vi "UI_AutoRefresh_Init.vi"(8 "error in (no error)":errorcluster, 10 "Parameters":T1={"Write TipStrips with details (T)"=TRUE, "Write Captions with UserLabels (T)"=TRUE, "Mode (ind only)"=enum."Indicators only"}, 11 "UI_Actor in":refnum<class "UI_Actor.lvclass">) -> (0 "error out":errorcluster, 3 "UI_Actor out":refnum<class "UI_Actor.lvclass">)   [LabVIEW 2020, in "UI_Actor.lvlib" / "UI_Actor.lvclass"]
uses:
  UI_Actor.lvclass
  ctl_AR_Parameters.ctl
  ctl_AR_Mode.ctl
  ctl_AR_Elmt.ctl
  UI_Actor.lvclass/UI_Actor.ctl
  UI_Actor Messages/UI_AutoRefresh_Init Msg/UI_AutoRefresh_Init Msg.lvclass/UI_AutoRefresh_Init Msg.ctl
  support/Actor Framework.lvlibp/1abvi3w/vi.lib/ActorFramework/Message Enqueuer/Enqueue.vi
  support/Databox.lvlibp/TypesTools/Config/Read System Label.vi
  UI_Actor Messages/UI_AutoRefresh_Init Msg/UI_AutoRefresh_Init Msg.lvclass
  support/Databox.lvlibp/TypesTools/Config/Config.lvclass
  support/Databox.lvlibp/TypesTools/Data/Data.lvclass
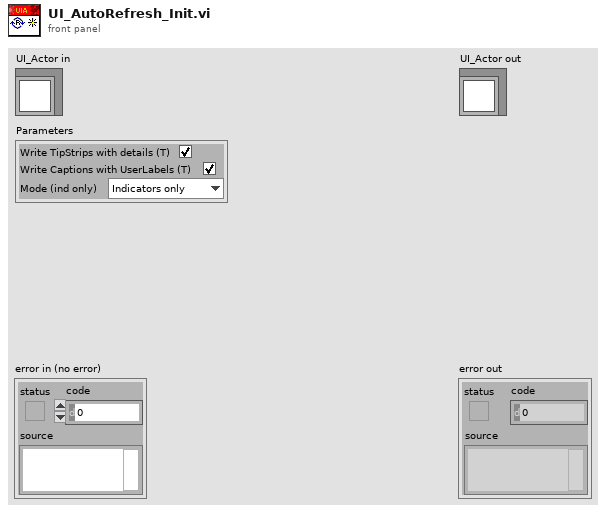
[diagram p1: front panel]
types:
  T1 = typedef "UI_Actor.lvlib/UI_Actor.lvclass/ctl_AR_Parameters.ctl" = cluster{"Write TipStrips with details (T)":bool, "Write Captions with UserLabels (T)":bool, "Mode (ind only)":T2}
  T2 = typedef "UI_Actor.lvlib/UI_Actor.lvclass/ctl_AR_Mode.ctl" = enum16{"Controls only", "Indicators only", "All"}
  T3 = typedef "UI_Actor.lvlib/UI_Actor.lvclass/ctl_AR_Elmt.ctl" = cluster{"AR by Index":bool, "Ref":refnum<vi>, "Index":i32, "Class ID":u32, "Sourcer":string, "SysLab":string}
  T4 = typedef "UI_Actor.lvlib/UI_Actor.lvclass/ctl_InternalMapItem.ctl" = cluster{"Config":refnum<class "Config.lvclass">, "LatestData":refnum<class "Data.lvclass">}
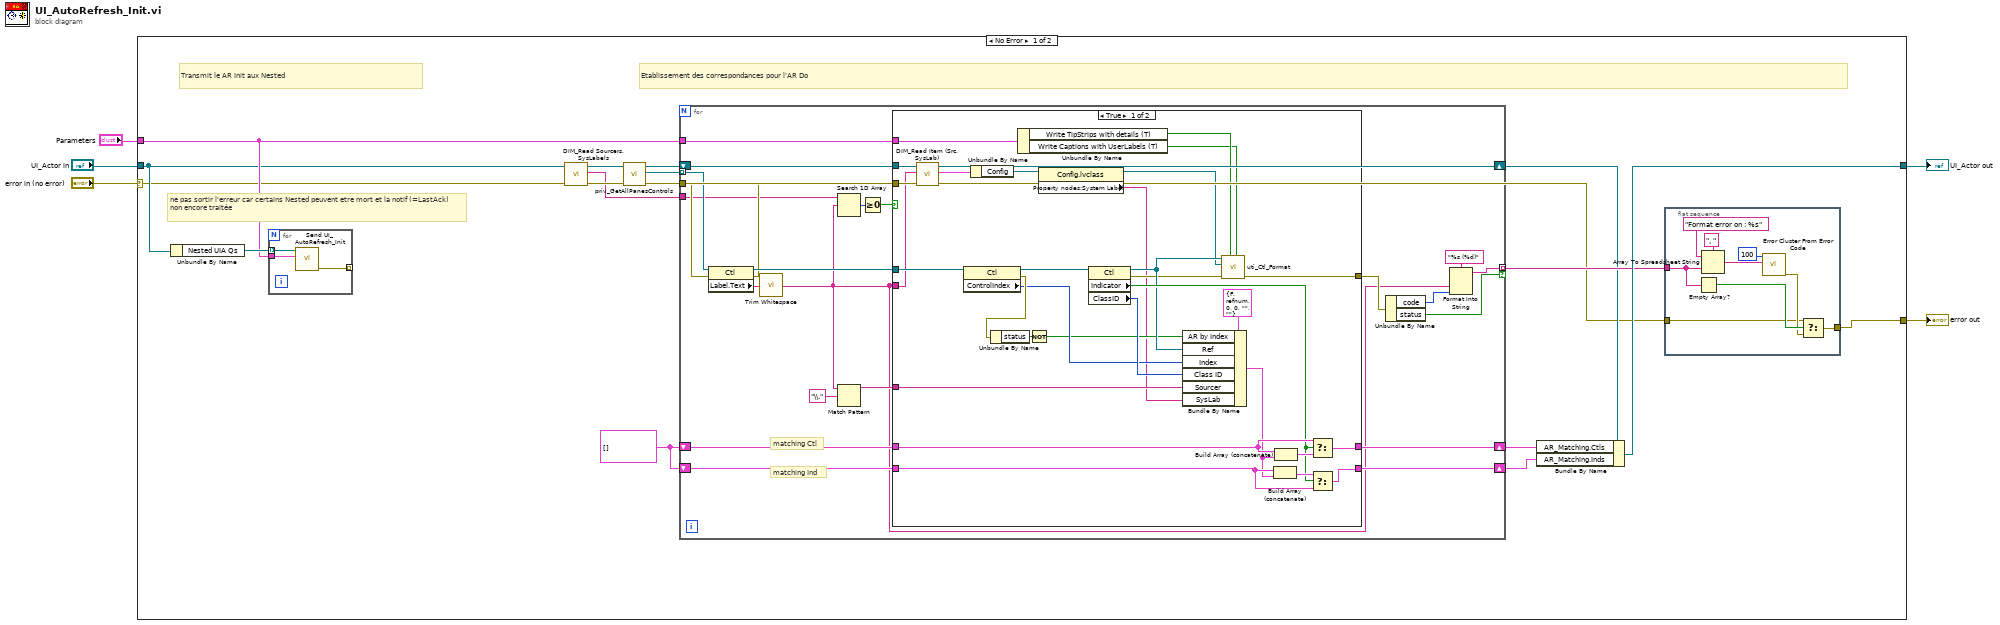
[diagram p0: block diagram]
diagram:
  n1 = case shown="No Error" "error in (no error)" {
    selector: "error in (no error)" -> [w8 w90]
    tunnel: [w22 w90] -> w1
    tunnel: [w21 w89] -> w3
    tunnel: "UI_Actor in" -> [w9 w89]
    tunnel: "Parameters" -> [w17 _]
    frame No Error {
      w16 = T3[] []
      # "ne pas sortir l'erreur car certains Nested peuvent etre mort et la notif (=LastAck) non encore traitée"
      # "Etablissement des correspondances pour l'AR Do"
      # "Transmit le AR Init aux Nested"
      n2 = Unbundle By Name(w9) -> ("Nested UIA Qs"=w18:refnum<class "Message Enqueuer.lvclass">[])
      n3 = for {
        tunnel: w17 -> [w88]
        tunnel: w18 -> [w87] mode=indexing
        tunnel: [w86] -> _ mode=indexing
        n4 = call "Send UI_AutoRefresh_Init.vi"("Parameters"=w88, "Message Enqueuer"=w87) -> ("error out"=w86:errorcluster)  [unwired: 8 in, 1 out]
      }
      n5 = call "DIM_Read Sourcers.SysLabels.vi"("error in (no error)"=w8, "UI_Actor in"=w9) -> ("error out"=w7:errorcluster, "DIM Sourcer.SysLabels"=w6:string[], "UI_Actor out"=w10:refnum<class "UI_Actor.lvclass">)  [unwired: 7 in]
      n6 = call "priv_GetAllPanesControls.vi"("error in (no error)"=w7, "UI_Actor in"=w10) -> ("error out"=w11:errorcluster, "Controls[]"=w19:refnum<vi>[], "UI_Actor out"=w13:refnum<class "UI_Actor.lvclass">)  [unwired: 7 in]
      n7 = for {
        tunnel: w19 -> [w44] mode=indexing
        shift-right: [w41] -> w14
        shift-left: w16 -> [w40]
        shift-right: [w38] -> w15
        shift-left: w16 -> [w39]
        tunnel: w17 -> [w36]
        tunnel: w11 -> [w43]
        tunnel: [w31] -> w20 mode=indexing if=w34
        shift-right: [w30] -> w12
        shift-left: w13 -> [w30]
        tunnel: w6 -> [w26]
        # "matching Ctl"
        # "matching Ind"
        n8 = property class="Ctl"(reference=w44, error in=w43) -> (reference out=w42:refnum<vi>, error out=w29:errorcluster, "Label.Text"=w37:string)
        n9 = call <vilib>:"Trim Whitespace.vi"("string"=w37) -> ("trimmed string"=w23:string)  [unwired: 1 in]
        n10 = Search 1D Array(1D array=w26, element=w23) -> (index of element=w25:i32)  [unwired: 1 in]
        n11 = Match Pattern(string=w23, regular expression="\\.") -> (before substring=w27:string)  [unwired: 1 in, 3 out]
        n12 = Greater Or Equal To 0?(x=w25) -> (x >= 0?=w24:bool)
        n13 = case shown="True" w24 {
          tunnel: w42 -> [w56 _]
          tunnel: [w67 w76] -> w41
          tunnel: w40 -> [w73 w76]
          tunnel: w39 -> [w72 w75]
          tunnel: [w69 w75] -> w38
          tunnel: [w64 _] -> w35
          tunnel: w36 -> [w63 _]
          tunnel: w29 -> [w48 _]
          tunnel: w27 -> [w50 _]
          tunnel: w30 -> [w47 _]
          tunnel: w23 -> [w45 _]
          frame True {
            n14 = call "DIM_Read Item (Src.SysLab).vi"("error in (no error)"=w48, "Sourcer.SysLabel"=w45, "UI_Actor in"=w47) -> ("DIM Item"=w46:T4)  [unwired: 5 in, 3 out]
            n15 = property class="Ctl"(reference=w56) -> (reference out=w57:refnum<vi>, error out=w58:errorcluster, "ControlIndex"=w52:i32)  [unwired: 1 in]
            n16 = Unbundle By Name(w46) -> ("Config"=w55:refnum<class "Config.lvclass">)
            n17 = Unbundle By Name(w58) -> ("status"=w60:bool)
            n18 = Unbundle By Name(w63) -> ("Write TipStrips with details (T)"=w62:bool, "Write Captions with UserLabels (T)"=w61:bool)
            n19 = Not(x=w60) -> (.not. x?=w51:bool)
            n20 = property class="Config.lvclass"(reference=w55) -> (reference out=w54:refnum<class "Config.lvclass">, "Property nodes:System Label"=w49:string)  [unwired: 1 in, 1 out]
            n21 = property class="Ctl"(reference=w57) -> (reference out=w65:refnum<vi>, error out=w59:errorcluster, "Indicator"=w66:bool, "ClassID"=w53:u32)  [unwired: 1 in]
            n22 = Bundle By Name(cluster=T3 {"AR by Index"=FALSE, "Ref"=refnum, "Index"=0, "Class ID"=0, "Sourcer"="", "SysLab"=""} ("AR_Elmt"), "AR by Index"=w51, "Ref"=w65, "Index"=w52, "Class ID"=w53, "Sourcer"=w50, "SysLab"=w49) -> (w70:T3)
            n23 = call "uti_Ctl_Format.vi"("Write Captions with UserLabels (T)"=w61, "Write TipStrips with details (T)"=w62, "error in (no error)"=w59, "Channel Config"=w54, "Control in"=w65) -> ("error out"=w64:errorcluster)  [unwired: 5 in, 1 out]
            n24 = Build Array (concatenate)(w72, w70) -> (w71:T3[])
            n25 = Build Array (concatenate)(w73, w70) -> (w68:T3[])
            n26 = Select(t=w73, s=w66, f=w68) -> (s? t:f=w67:T3[])
            n27 = Select(t=w71, s=w66, f=w72) -> (s? t:f=w69:T3[])
          }
          frame False {
          }
        }
        n28 = Unbundle By Name(w35) -> ("code"=w32:i32, "status"=w34:bool)
        n29 = Format Into String(format string="%s (%d)", w23, w32) -> (resulting string=w31:string)  [unwired: 2 in, 1 out]
      }
      n30 = Bundle By Name(cluster=w12, "AR_Matching.Ctls"=w14, "AR_Matching.Inds"=w15) -> (w21:refnum<class "UI_Actor.lvclass">)
      n31 = flat-sequence {
        tunnel: [w78] -> w22
        tunnel: w20 -> [w81]
        tunnel: w11 -> [w77]
        frame #0 {
          n32 = Empty Array?(array=w81) -> (empty?=w80:bool)
          n33 = Array To Spreadsheet String(delimiter (Tab)=", ", array=w81, 3:"Format error on : %s" ("error message (\"\")")) -> (spreadsheet string=w82:string)
          n34 = call <vilib>:"Error Cluster From Error Code.vi"("error message (\"\")"=w82, "error code (0)"=100) -> ("error out"=w79:errorcluster)  [unwired: 7 in]
          n35 = Select(t=w77, s=w80, f=w79) -> (s? t:f=w78:errorcluster)
        }
      }
    }
    frame Error {
    }
  }
  "error out" <- w1
  "UI_Actor out" <- w3
